vi "Write MERCANCIA.vi"(8 "error in (no error)":errorcluster, 10 "MERCANCIA":refnum<vi>, 11 "BD_CAFÉ_MXN_ENG in":refnum<class "BD_CAFÉ_MXN_ENG.lvclass">) -> (0 "error out":errorcluster, 3 "BD_CAFÉ_MXN_ENG out":refnum<class "BD_CAFÉ_MXN_ENG.lvclass">)   [LabVIEW 2019, in "BD_CAFÉ_MXN_ENG.lvlib" / "BD_CAFÉ_MXN_ENG.lvclass"]
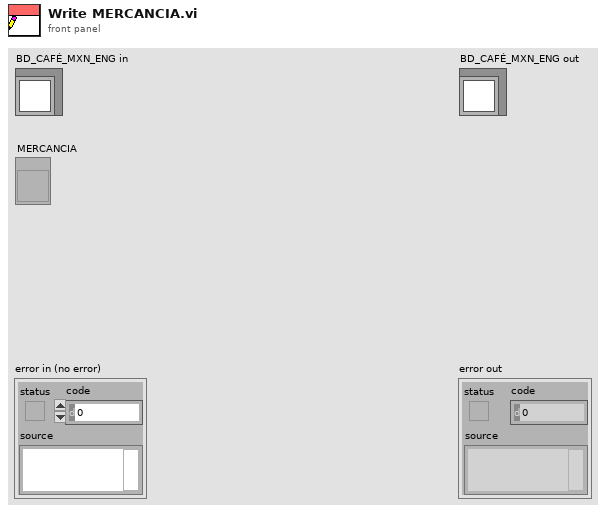
[diagram p1: front panel]
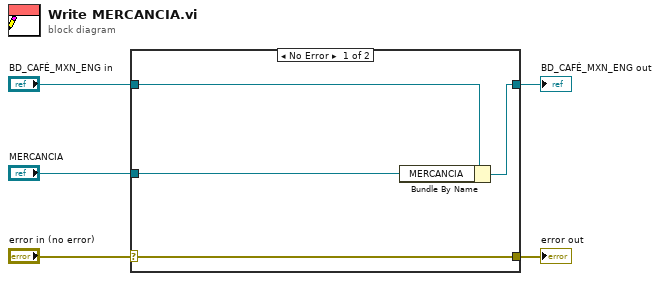
[diagram p0: block diagram]
diagram:
  n1 = case shown="No Error" "error in (no error)" {
    selector: "error in (no error)" -> [w9 w10]
    tunnel: [w9 w10] -> w4
    tunnel: [w7 w11] -> w2
    tunnel: "BD_CAFÉ_MXN_ENG in" -> [w8 w11]
    tunnel: "MERCANCIA" -> [w6 _]
    frame No Error {
      n2 = Bundle By Name(cluster=w8, "MERCANCIA"=w6) -> (w7:refnum<class "BD_CAFÉ_MXN_ENG.lvclass">)
    }
    frame Error {
    }
  }
  "error out" <- w4
  "BD_CAFÉ_MXN_ENG out" <- w2
